vi "Make DLL Param(Profile Rsp).vi"   [LabVIEW 2014, in "Keyence LJ-V7000.lvlib"]
uses:
  Keyence LJ-V7000.lvlib
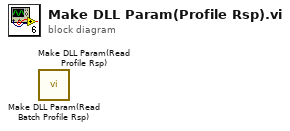
[diagram p0: block diagram]
diagram:
  n1 = call "Make DLL Param(Read Batch Profile Rsp).vi"() -> ()  [unwired: 1 in, 1 out]
  n2 = call "Make DLL Param(Read Profile Rsp).vi"() -> ()  [unwired: 1 in, 1 out]
